vi "Populate Device Names.vi"(8 "error in (no error)":errorcluster, 11 "RESOURCE NAME Ref":refnum<vi>) -> (0 "error out":errorcluster, 3 "RESOURCE NAME Ref out":refnum<vi>)   [LabVIEW 2025, in "I2C Bus Monitor UI.lvlib"]
uses:
  I2C Bus Monitor UI.lvlib
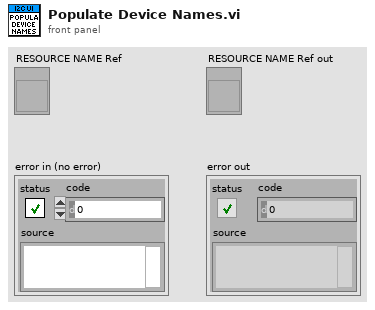
[diagram p1: front panel]
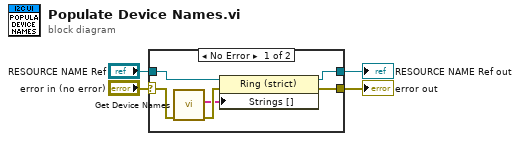
[diagram p0: block diagram]
diagram:
  n1 = case shown="No Error" "error in (no error)" {
    selector: "error in (no error)" -> [w7 w12]
    tunnel: "RESOURCE NAME Ref" -> [w9 w11]
    tunnel: [w6 w12] -> w2
    tunnel: [w5 w11] -> w1
    frame No Error {
      n2 = call "Get Device Names.vi"("error in (no error)"=w7) -> ("error out"=w10:errorcluster, "Alias"=w8:string[])  [unwired: 8 in, 1 out]
      n3 = property on="Property Node" class="Ring (strict)"(reference=w9, error in=w10, "Strings []"=w8) -> (reference out=w5:refnum<vi>, error out=w6:errorcluster)
    }
    frame Error {
    }
  }
  "error out" <- w2
  "RESOURCE NAME Ref out" <- w1
